vi "Drive Motor Recieve.vi"(10 "Drive Motor Handle In":T1, 11 "Error In":errorcluster) -> (2 "Drive Motor Handle Out":T1, 3 "Error Out":errorcluster)   [LabVIEW 2019]
uses:
  Drive Motor Handle.ctl
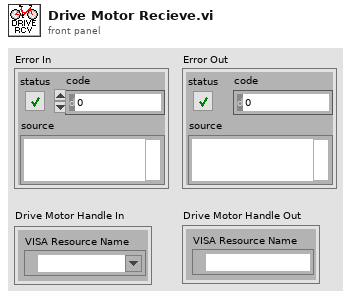
[diagram p1: front panel]
types:
  T1 = typedef "Drive Motor Handle.ctl" = cluster{"VISA Resource Name":refnum<visa-resource-name>}
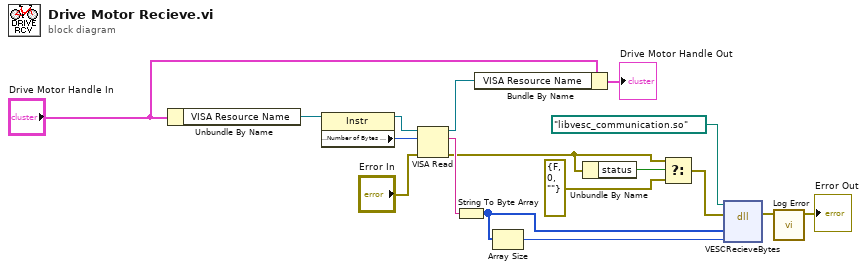
[diagram p0: block diagram]
diagram:
  n1 = Unbundle By Name("Drive Motor Handle In") -> ("VISA Resource Name"=w16:refnum<visa-resource-name>)
  n2 = property class="Instr"(reference=w16) -> (reference out=w8:refnum<visa-resource-name>, "Serial Settings:Number of Bytes at Serial Port"=w15:u32)  [unwired: 1 in, 1 out]
  n3 = VISA Read(VISA resource name=w8, byte count=w15, error in (no error)="Error In") -> (VISA resource name out=w10:refnum<visa-resource-name>, read buffer=w13:string, error out=w12:errorcluster)  [unwired: 1 out]
  n4 = String To Byte Array(string=w13) -> (unsigned byte array=w6:u8[])
  n5 = Bundle By Name(cluster="Drive Motor Handle In", "VISA Resource Name"=w10) -> (→"Drive Motor Handle Out":T1)
  n6 = Array Size(array=w6) -> (size(s)=w7:i32)
  n7 = Unbundle By Name(w12) -> ("status"=w4:bool)
  n8 = Select(t=w12, s=w4, f=errorcluster {"status"=FALSE, "code"=0, "source"=""}) -> (s? t:f=w3:errorcluster)
  n9 = dll-call lib="?" fn="VESCRecieveBytes"(path in=path "libvesc_communication.so", error in=w3, "bytes"=w6, "length"=w7) -> (error out=w1:errorcluster)  [unwired: 4 in, 1 out]
  n10 = call "Log Error.vi"("Error In"=w1) -> ("Error Out"=→"Error Out":errorcluster)  [unwired: 10 in]
